vi "Encoder Slowdown.vi"(9 "Threshold":dbl, 10 "Speed":dbl(slide) scale=0.0..10.0) -> (2 "Motor stalling?":bool)   [LabVIEW 2015]
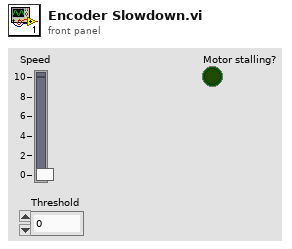
[diagram p1: front panel]
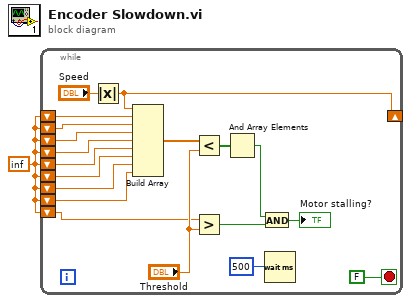
[diagram p0: block diagram]
diagram:
  w1 = inf
  n1 = while {
    shift-right: [w5] -> _
    shift-left: w1 -> [w20]
    shift-left: w1 -> [w19]
    shift-left: w1 -> [w18]
    shift-left: w1 -> [w17]
    shift-left: w1 -> [w16]
    shift-left: w1 -> [w15]
    shift-left: w1 -> [w14]
    shift-left: w1 -> [w13]
    shift-left: w1 -> [w3]
    stop <- FALSE stop-if-true
    n2 = Absolute Value(x="Speed") -> (abs(x)=w5:dbl)
    n3 = Build Array(w5, w20, w19, w18, w17, w16, w15, w14, w13) -> (w4:dbl[])
    n4 = Less?(x=w4, y="Threshold") -> (x < y?=w11:bool[])
    n5 = Greater?(x=w3, y="Threshold") -> (0:w9:bool)
    n6 = And Array Elements(Boolean array=w11) -> (logical AND=w10:bool)
    n7 = And(x=w10, y=w9) -> (x .and. y?=→"Motor stalling?":bool)
    n8 = Wait (ms)(milliseconds to wait=u32 500) -> ()  [unwired: 1 out]
  }
